vi "00 Main (single phase) (x64-2018).vi"() -> ()   [LabVIEW 2017]
uses:
  OpenPMU_V1/OpenPMU_V1/SourceCode/Control 1.ctl
  <vilib>/DAQmx/read.llb/DAQmx Read (Analog 1D Wfm NChan NSamp).vi
  <vilib>/DAQmx/miscellaneous.llb/DAQmx Fill In Error Info.vi
panel:
  out "Waveform Graph":waveform(dbl)[](graph)
  out "error out":errorcluster
  in  "DAQmx Task Name":refnum<k21>
  out "Error out (DAQ Loop)":errorcluster
  out "DAQ Loop Iterations":i32
  out "Raw DAQ Output":dynamicdata(graph)=[{"t0"=timestamp(3367839419.335167 s since 1904-01-01), "dt"=0.00016666666666666663, "Y"=array[240 elements], "attributes"=variant("NI_ChannelName"=variant(string "Voltage_0"), "NI_UnitDescription"=variant(string "Volts"))}, {"t0"=timestamp(3367839419.3351874 s since 1904-01-01), "dt"=0.00016666666666666663, "Y"=array[240 elements], "attributes"=variant("NI_ChannelName"=variant(string "Voltage_1"), "NI_UnitDescription"=variant(string "Volts"))}, {"t0"=timestamp(3367839419.3352084 s since 1904-01-01), "dt"=0.00016666666666666663, "Y"=array[240 elements], "attributes"=variant("NI_ChannelName"=variant(string "Voltage_2"), "NI_UnitDescription"=variant(string "Volts"))}]
  in  "All Stop!":bool
  out "Frequency":dynamicdata(graph)
  out "Phase":dynamicdata(graph) caption="Frequency"
  out "Frequency":dbl format="%.2f"
  out "Amplitude":dbl format="%.2f"
  out "Phase":dbl format="%.2f"
  out "Acquisition Time":timestamp
  out "Voltage Waveform":T1=[{"t0"=timestamp(3377170241.8512917 s since 1904-01-01), "dt"=0.00016666666666666663, "Y"=array[300 elements]}, {"t0"=timestamp(3377170241.8513126 s since 1904-01-01), "dt"=0.00016666666666666663, "Y"=array[300 elements]}, {"t0"=timestamp(3377170241.8513336 s since 1904-01-01), "dt"=0.00016666666666666663, "Y"=array[300 elements]}]
  out "IP":string
  out "Port":i32
  out "Transmitted Data":string
  out "Stop":bool
  out "Elements in Acquisition Buffer":i32
  # "V1.2 - PFI0 (Single Phase)"
  # "50.5"
  # "The code and design of this VI are licensed \nunder the terms of the New BSD License.\nPlease see the VI documentation or License.txt\nfor more details.\n\nCopyright (c) 2012, David Laverty\nwww.OpenPMU.org"
  # "Configuration Information:\n\nThe ID and IP address to which the OpenPMU sends data is configured by 'C:\\PMUconfig.ini'.  If this doesn't exist, create it.\n\nCopy and paste the blue text below without the dashed lines into PMUconfig.ini.\n\n[Telecoms]\nID=PMU123\nIP=192.168.1.100\nPort=40001\n\nIP and Port may be any values within normal IPv4 range.  ID should be six alpha-numeric characters."
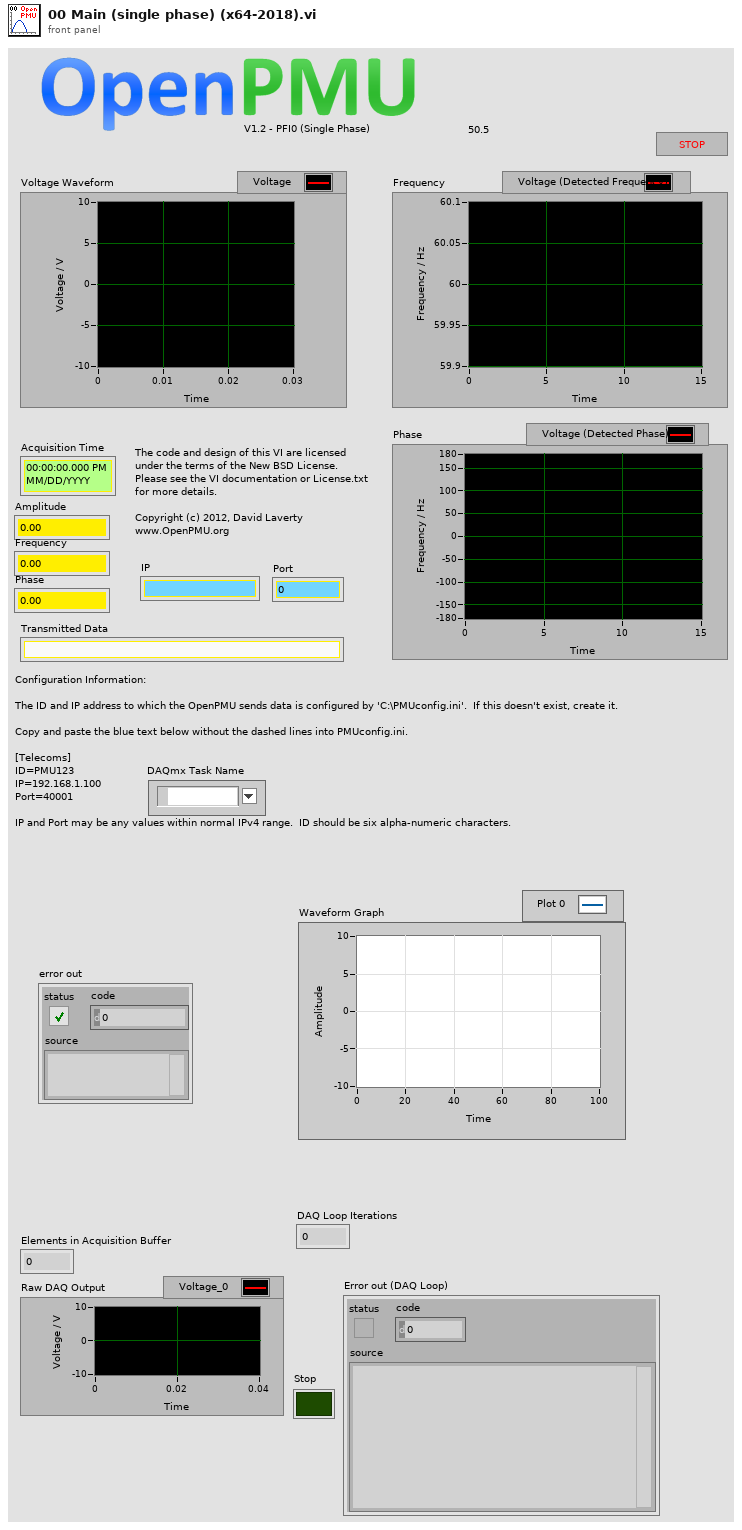
[diagram p1: front panel]
types:
  T1 = typedef "Control 1.ctl" = dynamicdata
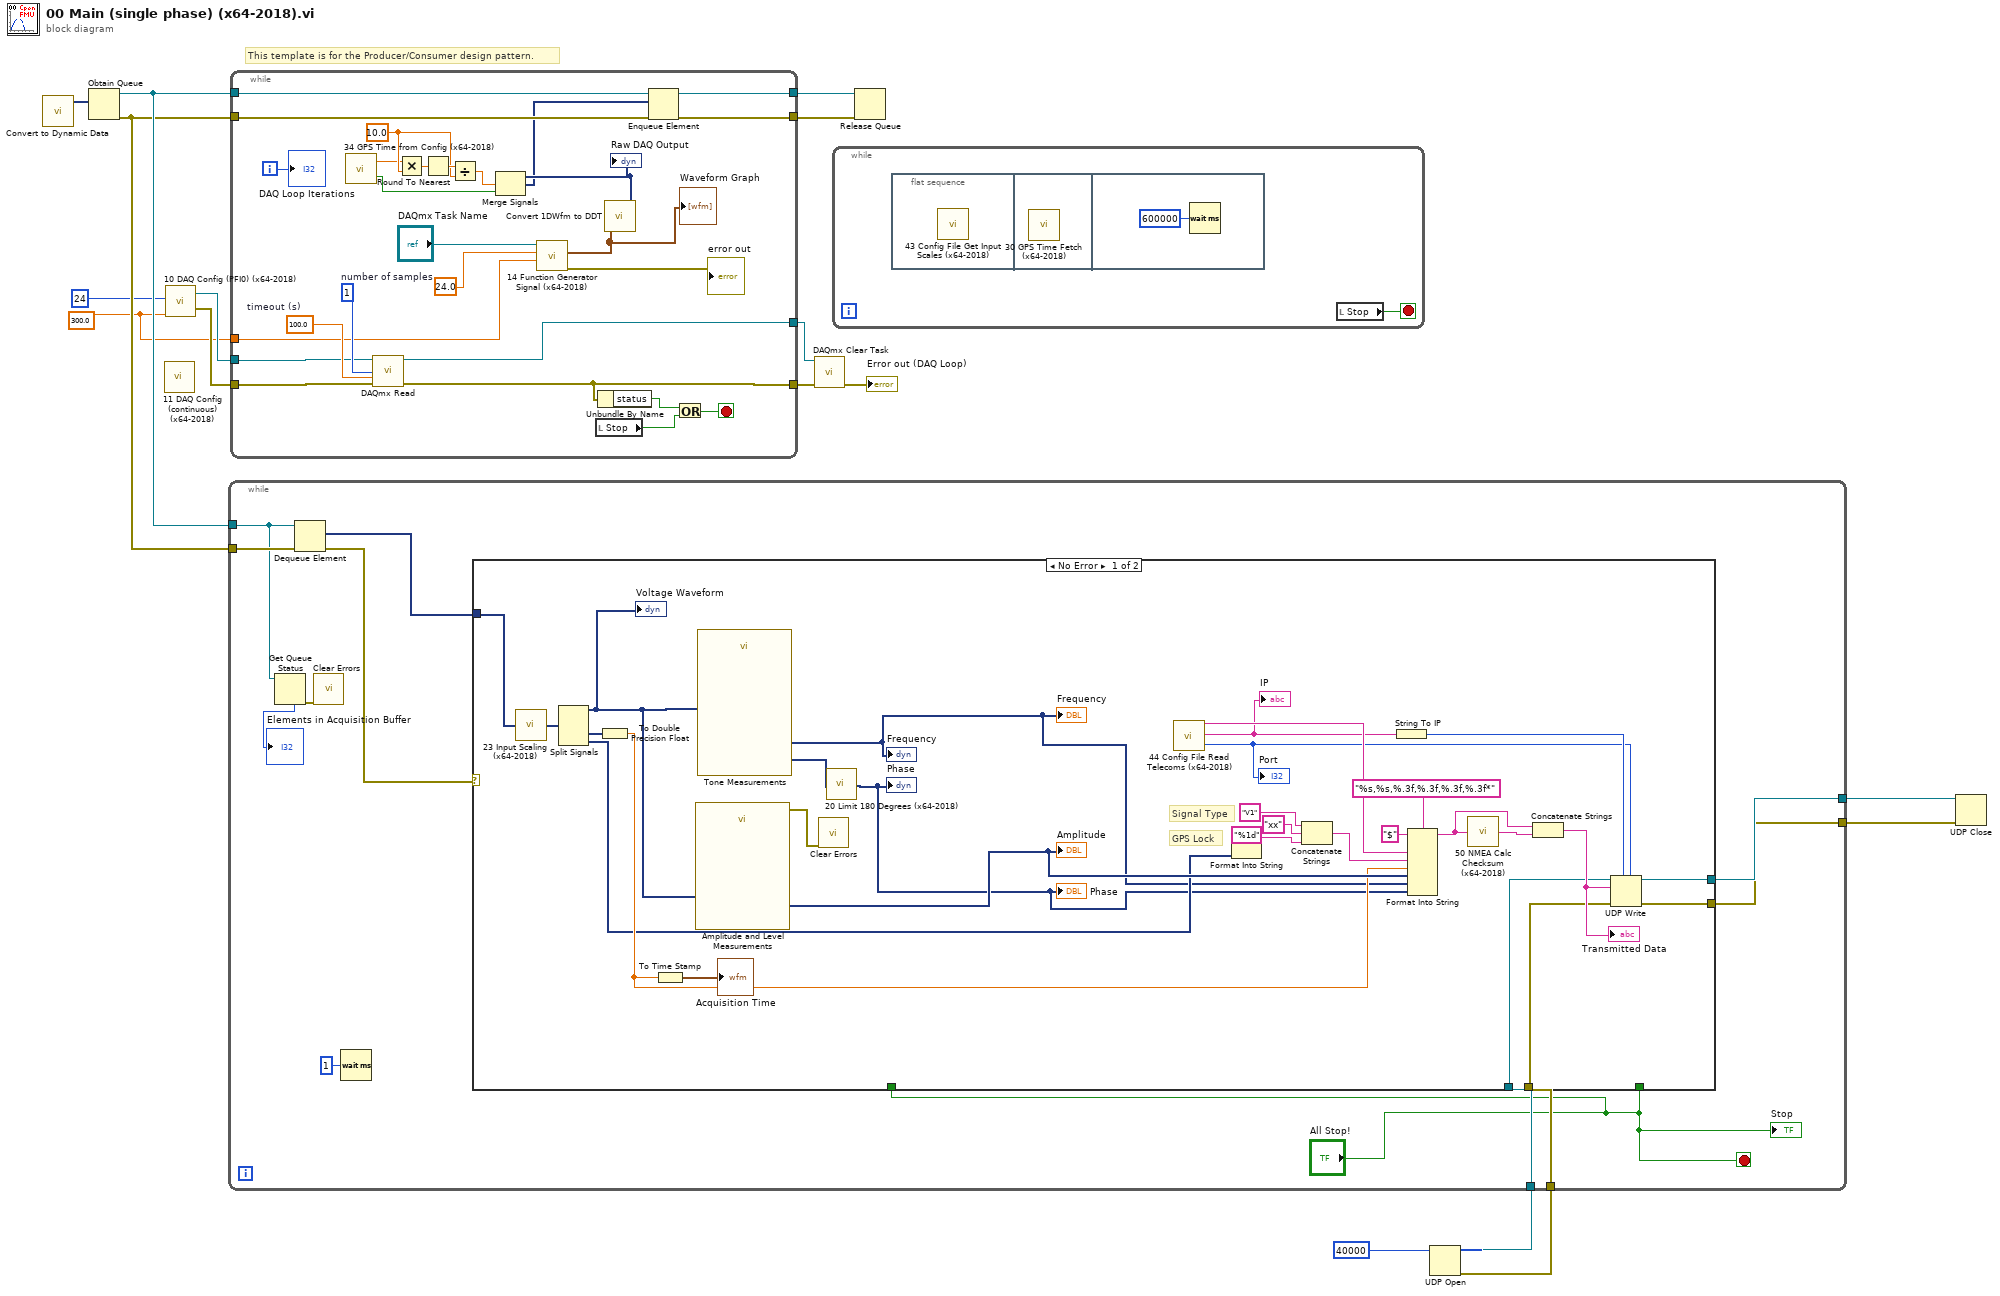
[diagram p0: block diagram]
diagram:
  w1 = 300.0 ("rate")
  # "This template is for the Producer/Consumer design pattern."
  n1 = call "Convert to Dynamic Data"() -> ("Dynamic Data Type"=w14:dynamicdata)  [unwired: 4 in]
  n2 = Obtain Queue(element data type=w14) -> (queue out=w11:refnum<queue>, error out=w10:errorcluster)  [unwired: 4 in, 1 out]
  n3 = call "11 DAQ Config (continuous) (x64-2018).vi"() -> ()  [unwired: 1 in, 2 out]
  n4 = call "10 DAQ Config (PFI0) (x64-2018).vi"("rate"=w1, "number of samples"=24) -> ("Error Out"=w2:errorcluster, "task out"=w3:refnum<k21>)  [unwired: 1 in]
  n5 = while {
    tunnel: w2 -> [w32]
    tunnel: w3 -> [w33]
    tunnel: [w41] -> w17
    tunnel: [w20] -> w16
    tunnel: w11 -> [w37]
    tunnel: w10 -> [w36]
    tunnel: [w35] -> w13
    tunnel: [w34] -> w12
    tunnel: w1 -> [w21]
    i -> [w40]
    stop <- w39 stop-if-true
    w26 = 10.0 ("y")
    w42 = 100.0  # timeout (s)
    w44 = 1  # number of samples
    n6 = call "34 GPS Time from Config (x64-2018).vi"() -> ("GPS Lock"=w24:bool, "Time"=w25:dbl)  [unwired: 2 in]
    n7 = call-poly <vilib>:"DAQmx Read.vi"("task/channels in"=w33, "number of samples per channel"=w44, "timeout"=w42, "error in"=w32) -> ("task out"=w41:refnum<k21>, "error out"=w20:errorcluster)  [unwired: 9 in, 1 out]
    n8 = Multiply(x=w25, y=w26) -> (x*y=w29:dbl)
    n9 = Round To Nearest(number=w29) -> (nearest integer value=w28:dbl)
    n10 = Divide(x=w28, y=w26) -> (x/y=w27:dbl)
    n11 = call "14 Function Generator Signal (x64-2018).vi"("Rate"=w21, "Number of samples per channel"=24.0 ("rate"), "task/channels in"="DAQmx Task Name") -> ("Error Out"=→"error out":errorcluster, "data"=w18:waveform(dbl)[])  [unwired: 6 in, 1 out]
    "Waveform Graph" <- w18
    n12 = local read "Stop"() -> (w38:bool)
    n13 = Unbundle By Name(w20) -> ("status"=w43:bool)
    n14 = call <vilib>:"Convert 1DWfm to DDT.vi"("Array of Waveforms"=w18) -> ("Dynamic Data Type"=w31:dynamicdata)  [unwired: 3 in]
    "Raw DAQ Output" <- w31
    n15 = Merge Signals(w31, w27, w24) -> (w30:dynamicdata)
    n16 = Enqueue Element(queue=w37, element=w30, error in (no error)=w36) -> (queue out=w35:refnum<queue>, error out=w34:errorcluster)  [unwired: 1 in, 1 out]
    n17 = Or(x=w43, y=w38) -> (x .or. y?=w39:bool)
    "DAQ Loop Iterations" <- w40
  }
  n18 = call <vilib>:"DAQmx Clear Task.vi"("task in"=w17, "error in"=w16) -> ("error out"=→"Error out (DAQ Loop)":errorcluster)  [unwired: 13 in]
  n19 = while {
    stop <- w45 stop-if-true
    n20 = flat-sequence {
      frame #0 {
        n21 = call "43 Config File Get Input Scales (x64-2018).vi"() -> ()  [unwired: 1 in]
      }
      frame #1 {
        n22 = call "30 GPS Time Fetch (x64-2018).vi"() -> ()  [unwired: 1 in]
      }
      frame #2 {
        n23 = Wait (ms)(milliseconds to wait=u32 600000) -> ()  [unwired: 1 out]
      }
    }
    n24 = local read "Stop"() -> (w45:bool)
  }
  n25 = Release Queue(queue=w13, error in (no error)=w12) -> ()  [unwired: 1 in, 3 out]
  n26 = UDP Open(11:u16 40000 ("port")) -> (port=w8:refnum<k16>, 0:w7:errorcluster)  [unwired: 4 in, 1 out]
  n27 = while {
    tunnel: w11 -> [w53]
    tunnel: w10 -> [w55]
    tunnel: w8 -> [w52]
    tunnel: w7 -> [w51]
    tunnel: [w50] -> w6
    tunnel: [w49] -> w5
    stop <- "All Stop!" stop-if-true
    n28 = Get Queue Status(queue=w53) -> (error out=w48:errorcluster, # elements in queue=→"Elements in Acquisition Buffer":i32)  [unwired: 2 in, 6 out]
    n29 = Dequeue Element(queue=w53, error in (no error)=w55) -> (element=w56:dynamicdata, error out=w57:errorcluster)  [unwired: 1 in, 2 out]
    n30 = call <vilib>:"Clear Errors.vi"("error in (no error)"=w48) -> ()  [unwired: 5 in, 2 out]
    n31 = Wait (ms)(milliseconds to wait=u32 1) -> ()  [unwired: 1 out]
    n32 = case shown="No Error" w57 {
      tunnel: w56 -> [w69 _]
      tunnel: w52 -> [w82 w90]
      tunnel: w51 -> [w81 w89]
      tunnel: [w80 w90] -> w50
      tunnel: [w79 w89] -> w49
      tunnel: "All Stop!" -> [_ _]
      tunnel: "All Stop!" -> [_ _]
      frame No Error {
        # "GPS Lock"
        # "Signal Type"
        n33 = call "23 Input Scaling (x64-2018).vi"("Input (Raw)"=w69) -> ("Output (Scaled)"=w68:dynamicdata)
        n34 = Split Signals(w68) -> (w59:dynamicdata, w78:dynamicdata, w75:dynamicdata)  [unwired: 5 in, 2 out]
        "Voltage Waveform" <- w59
        n35 = To Double Precision Float(number=w78) -> (double precision float=w76:dbl)
        n36 = To Time Stamp(1:w76) -> (0:→"Acquisition Time":timestamp)
        n37 = call "Amplitude and Level Measurements"("Signals"=w59) -> ("Cycle RMS"=w77:dynamicdata, "error out"=w88:errorcluster)  [unwired: 13 in]
        "Amplitude" <- w77
        n38 = call "Tone Measurements"("Signals"=w59) -> ("Phase"=w67:dynamicdata, "Frequency"=w61:dynamicdata)  [unwired: 7 in, 2 out]
        "Frequency" <- w61
        "Frequency" <- w61
        n39 = call <vilib>:"Clear Errors.vi"("error in (no error)"=w88) -> ()  [unwired: 5 in, 2 out]
        n40 = call "20 Limit 180 Degrees (x64-2018).vi"("Angle In"=w67) -> ("Angle Out"=w60:dynamicdata)
        "Phase" <- w60
        "Phase" <- w60
        n41 = call "44 Config File Read Telecoms (x64-2018).vi"() -> ("Port"=w64:i32, "IP"=w65:string, "ID"=w66:string)  [unwired: 3 in]
        "IP" <- w65
        "Port" <- w64
        n42 = Format Into String(format string="%1d", w75) -> (resulting string=w70:string)  [unwired: 2 in, 1 out]
        n43 = Concatenate Strings("V1" ("input 2"), "xx" ("string"), w70) -> (w72:string)
        n44 = String To IP(1:w65) -> (0:w84:u32)
        n45 = Format Into String(format string="%s,%s,%.3f,%.3f,%.3f,%.3f*", initial string="$", w66, w72, w76, w77, w61, w60) -> (resulting string=w63:string)  [unwired: 1 in, 1 out]
        n46 = call "50 NMEA Calc Checksum (x64-2018).vi"("GPS String"=w63) -> ("hex integer string"=w62:string)  [unwired: 1 in, 1 out]
        n47 = Concatenate Strings(w63, w62) -> (w83:string)
        "Transmitted Data" <- w83
        n48 = UDP Write(address=w84, port or service name=w64, connection ID=w82, data in=w83, 8:w81) -> (error out=w79:errorcluster, 3:w80:refnum<k16>)  [unwired: 1 in]
      }
      frame Error {
      }
    }
    "Stop" <- "All Stop!"
  }
  n49 = UDP Close(connection ID=w6, 8:w5) -> ()  [unwired: 2 out]
